vi "电磁阀准备.vi"() -> ()   [LabVIEW 2013]
panel:
  in  "电磁阀准备":bool
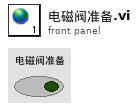
[diagram p1: front panel]
diagram:
